vi "test coerce and update 1.vi"() -> ()   [LabVIEW 2020]
panel:
  out "Value":dbl
  in  "max":dbl
  in  "min":dbl
  in  "stop":bool
  in  "tested":dbl
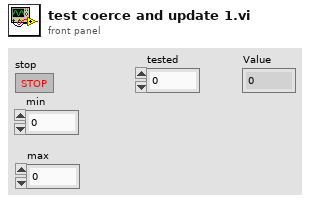
[diagram p1: front panel]
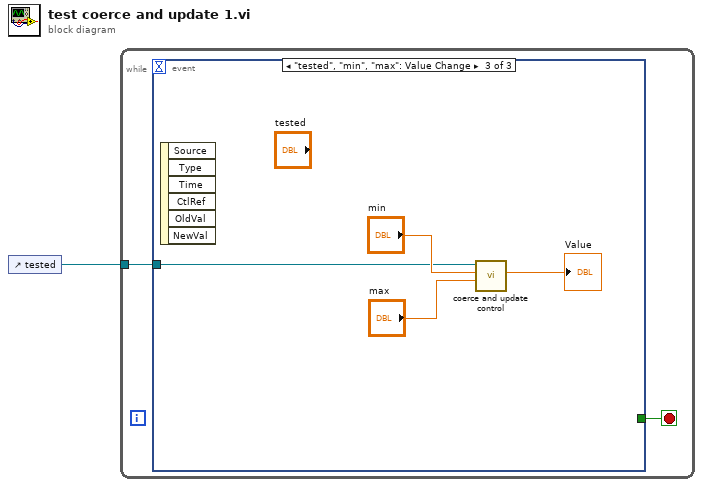
[diagram p0: block diagram]
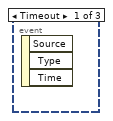
[diagram p2: hidden frame]
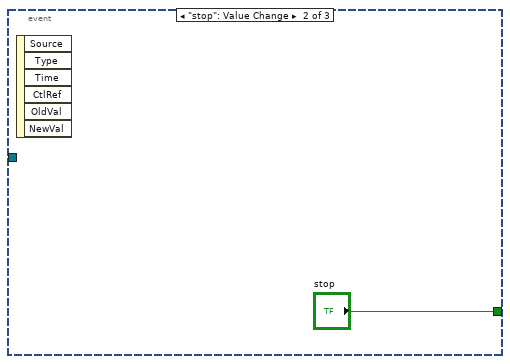
[diagram p3: hidden frame]
diagram:
  n1 = control-ref of="tested"() -> (w1:refnum<vi>)
  n2 = while {
    tunnel: w1 -> [w2]
    stop <- w3 stop-if-true
    n3 = event shown="[2] \"tested\", \"min\", \"max\": Value Change" {
      selector: _ -> [_ _ _]
      dyn-events: _ -> [_ _ _]
      timeout: _ -> [_ _ _]
      tunnel: [_ "stop" _] -> w3
      tunnel: w2 -> [_ _ w6]
      event Timeout {
        n4 = event-data() -> ()  [unwired: 1 in, 3 out]
      }
      event "stop": Value Change {
        n5 = event-data() -> ()  [unwired: 1 in, 6 out]
      }
      event "tested", "min", "max": Value Change {
        n6 = event-data() -> ()  [unwired: 1 in, 6 out]
        n7 = call "coerce and update control.vi"("max"="max", "min"="min", "Refnum In"=w6) -> ("Value"=→"Value":dbl)  [unwired: 6 in, 2 out]
      }
    }
  }
